vi "SetState.vi"(0 "reference in":refnum<class "Device.lvclass">, 5 "State":u16, 11 "error in (no error)":errorcluster) -> (4 "reference out":refnum<class "Device.lvclass">, 15 "error out":errorcluster)   [LabVIEW 2019]
uses:
  Device.lvclass
  D:/H4000/src/Proccess_class/Proccess.lvclass
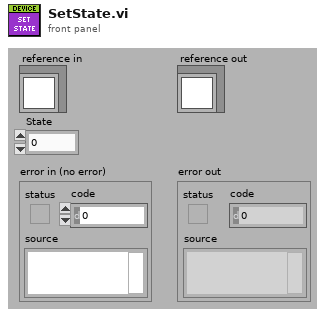
[diagram p1: front panel]
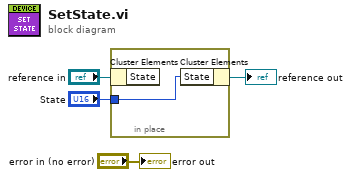
[diagram p0: block diagram]
diagram:
  n1 = in-place {
    in-place-border: "State" -> [w5]
    n2 = in-place-cluster #1("reference in") -> ()  [unwired: 1 out]
    n3 = in-place-cluster #1("State"=w5) -> (→"reference out":refnum<class "Device.lvclass">)
  }
  "error out" <- "error in (no error)"
